vi "TGFrogFINAL.vi"() -> ()   [LabVIEW 2013]
uses:
  <vilib>/Analysis/2dsp.llb/Complex FFT.vi
  <vilib>/Analysis/2dsp.llb/Inverse Complex FFT.vi
  <vilib>/Analysis/NI_AALPro.lvlib
panel:
  out "Error":dbl(graph)
  out "Stationary Solution":bool
  out "Current Error":dbl
  out "Target Error":dbl
  out "size(s) 3":i32
  out "size(s) 2":i32[](array[numeric])
  out "element 2":i32
  in  "Max Iterations":i32
  out "Numeric":i32
  out "element":i32
  out "Experiment Trace":dbl[][](graph)
  out "size(s)":i32[](array[numeric])
  in  "PG Test Data":dbl[][](array[numeric])=array129x256[33024 elements]
  in  "Beta":dbl(slide) scale=-0.01..0.01
  in  "Omega":dbl(slide) scale=0.0..0.5
  in  "Tau":dbl(slide) scale=0.0..100.0
  out "Electric Field":dbl[][](graph)
  out "Recovered Trace":dbl[][](graph)
  out "Gating Visualize":dbl[][](graph)
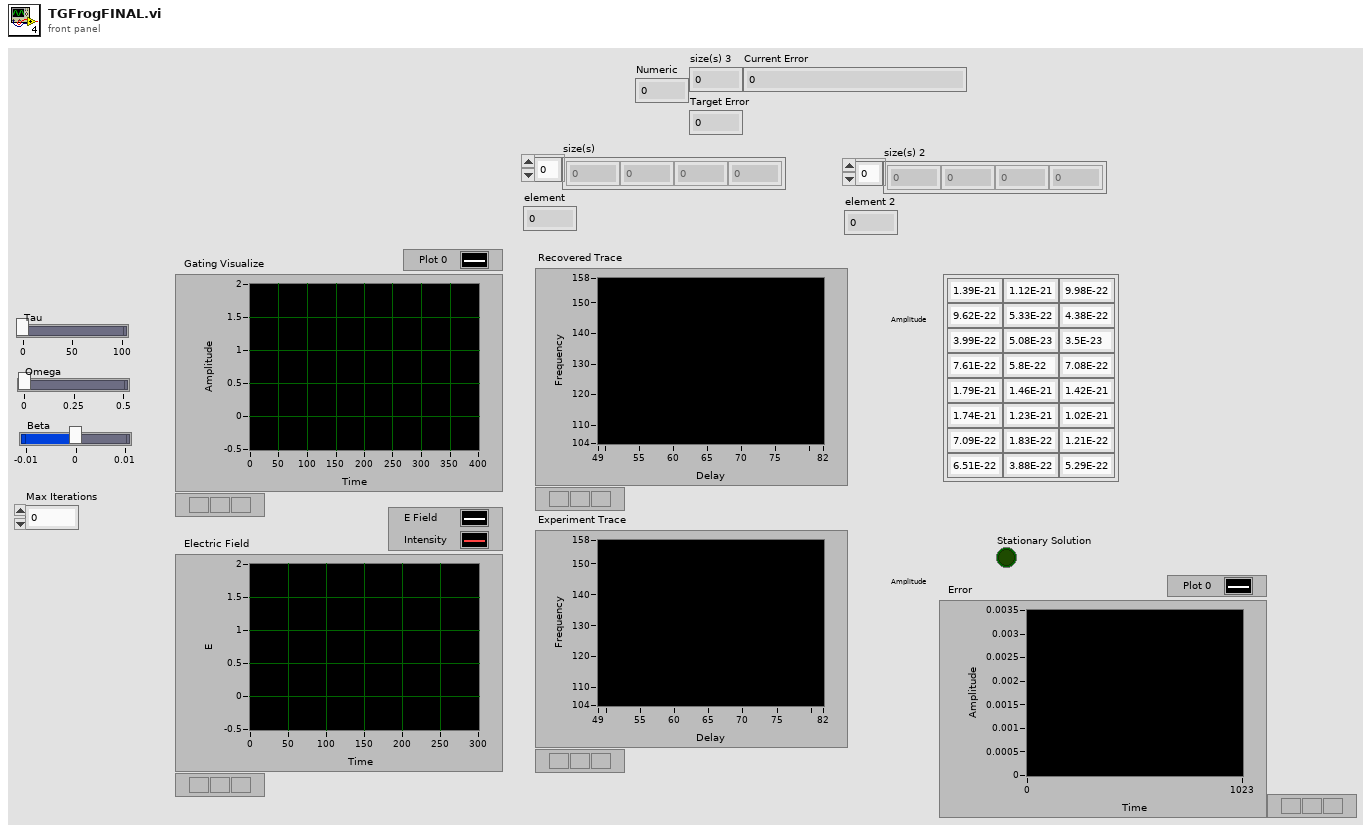
[diagram p1: front panel]
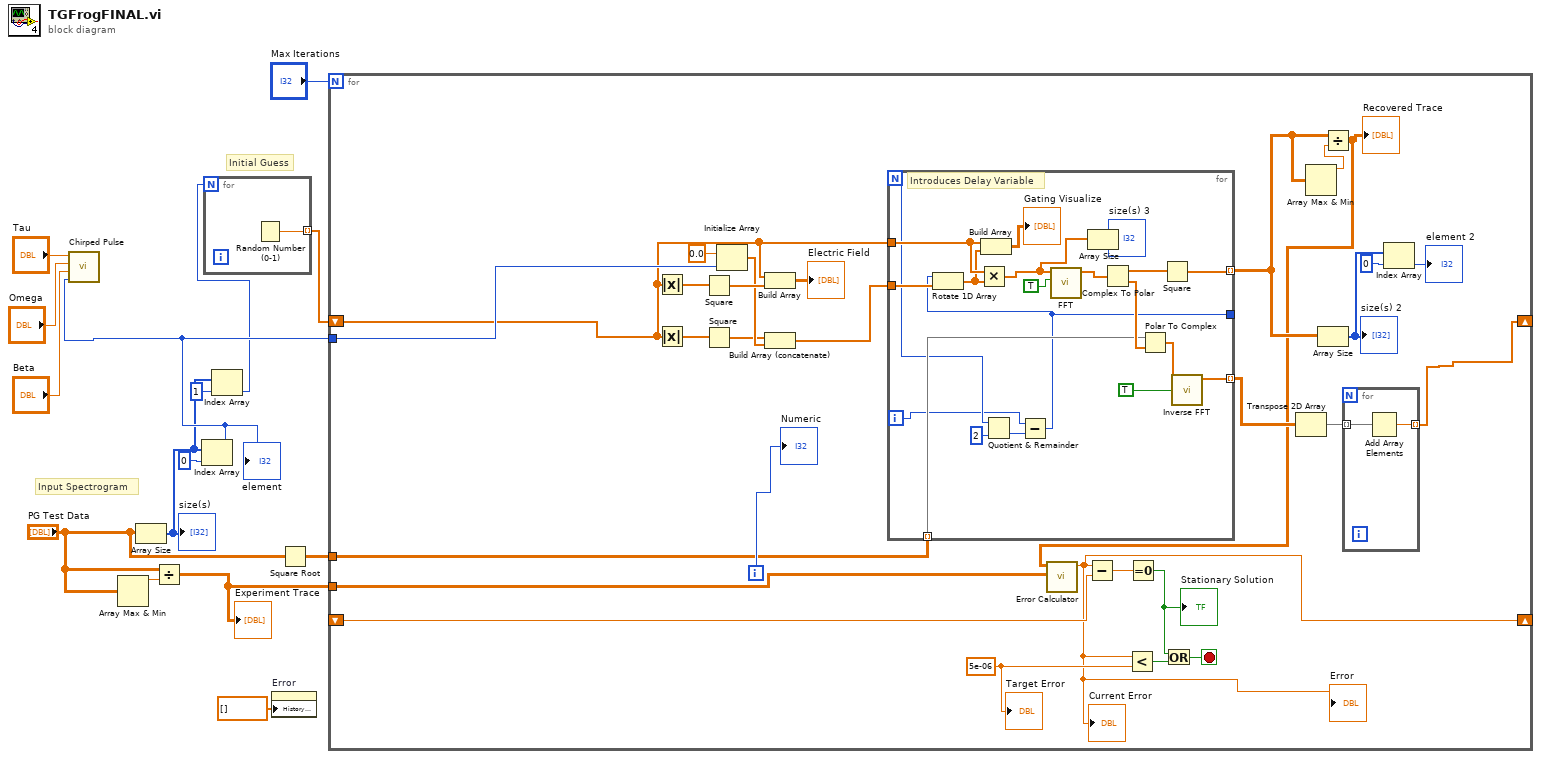
[diagram p0: block diagram]
diagram:
  # "Initial Guess"
  # "Input Spectrogram"
  n1 = Array Max & Min(array="PG Test Data") -> (max value=w7:dbl)  [unwired: 3 out]
  n2 = Array Size(array="PG Test Data") -> (size(s)=w5:i32[])
  "size(s)" <- w5
  n3 = Divide(x="PG Test Data", y=w7) -> (x/y=w2:dbl[][])
  "Experiment Trace" <- w2
  n4 = Index Array(array=w5, index=0) -> (element=w9:i32)
  "element" <- w9
  n5 = call "Chirped Pulse.vi"("Numeric"=w9, "Beta"="Beta", "Omega"="Omega", "Tau"="Tau") -> ()  [unwired: 6 in, 2 out]
  n6 = Index Array(array=w5, index=1) -> (element=w3:i32)
  n7 = for {
    N: w3 -> [_]
    tunnel: [w16] -> w8 mode=indexing
    n8 = Random Number (0-1)() -> (number: 0 to 1=w16:dbl)
  }
  n9 = property on="Error" class="WFChart (strict)"("History Data"=dbl[] []) -> ()  [unwired: 2 in, 2 out]
  n10 = Square Root(x="PG Test Data") -> (sqrt(x)=w10:dbl[][])
  n11 = for {
    N: "Max Iterations" -> [_]
    tunnel: w10 -> [w26]
    tunnel: w9 -> [w37]
    shift-right: [w28] -> _
    shift-left: w8 -> [w30]
    shift-right: [w17] -> _
    shift-left: _ -> [w22]
    tunnel: w2 -> [w19]
    i -> [w45]
    stop <- w24 stop-if-true
    w23 = 5e-06 ("y")
    n12 = Absolute Value(x=w30) -> (abs(x)=w42:dbl[])
    n13 = Absolute Value(x=w30) -> (abs(x)=w39:dbl[])
    n14 = Square(x=w42) -> (x^2=w43:dbl[])
    n15 = Square(x=w39) -> (x^2=w40:dbl[])
    n16 = Initialize Array(0.0 ("element"), w37) -> (w41:dbl[])
    n17 = Build Array(w30, w43) -> (→"Electric Field":cdb[][])
    n18 = Build Array (concatenate)(w40, w41) -> (w29:dbl[])
    n19 = for {
      N -> [w56]
      tunnel: w30 -> [w66]
      tunnel: w29 -> [w67]
      tunnel: [w51] -> w27 mode=indexing
      tunnel: w26 -> [w62] mode=indexing
      tunnel: [w59] -> w32 mode=indexing
      tunnel: [w54] -> _
      i -> [w55]
      # "Introduces Delay Variable"
      n20 = Quotient & Remainder(x=w56, y=2) -> (floor(x/y)=w57:i32)  [unwired: 1 out]
      n21 = Subtract(x=w55, y=w57) -> (x-y=w54:i32)
      n22 = Rotate 1D Array(1:w67, 2:w54) -> (0:w49:dbl[])
      n23 = Multiply(x=w66, y=w49) -> (x*y=w48:cdb[])
      n24 = Build Array(w66, w49) -> (→"Gating Visualize":cdb[][])
      n25 = call-poly <vilib>:"FFT.vi"("shift?"=TRUE, "X"=w48) -> ("FFT {X}"=w53:cdb[])  [unwired: 8 in, 1 out]
      n26 = Array Size(array=w48) -> (size(s)=→"size(s) 3":i32)
      n27 = Complex To Polar(r * e^(i*theta)=w53) -> (r=w64:dbl[], theta=w63:dbl[])
      n28 = Polar To Complex(1:w63, 2:w62) -> (0:w61:cdb[])
      n29 = Square(x=w64) -> (x^2=w51:dbl[])
      n30 = call-poly <vilib>:"Inverse FFT.vi"("shift?"=TRUE, "FFT {X}"=w61) -> ("X"=w59:cdb[])  [unwired: 8 in, 1 out]
    }
    n31 = Transpose 2D Array(2D array=w32) -> (transposed array=w33:cdb[][])
    n32 = Array Max & Min(array=w27) -> (max value=w31:dbl)  [unwired: 3 out]
    n33 = Array Size(array=w27) -> (size(s)=w34:i32[])
    "size(s) 2" <- w34
    n34 = Divide(x=w27, y=w31) -> (x/y=w18:dbl[][])
    "Recovered Trace" <- w18
    n35 = call "Error Calculator.vi"("Recovered Trace"=w18, "Experiment Trace"=w19) -> ("Current Error"=w17:dbl)  [unwired: 8 in]
    "Current Error" <- w17
    "Error" <- w17
    n36 = Subtract(x=w17, y=w22) -> (x-y=w20:dbl)
    n37 = Less?(x=w17, y=w23) -> (x < y?=w25:bool)
    n38 = Equal To 0?(x=w20) -> (x = 0?=w21:bool)
    "Stationary Solution" <- w21
    n39 = Or(x=w21, y=w25) -> (x .or. y?=w24:bool)
    n40 = for {
      tunnel: w33 -> [w46] mode=indexing
      tunnel: [w47] -> w28 mode=indexing
      n41 = Add Array Elements(numeric array=w46) -> (sum=w47:cdb)
    }
    n42 = Index Array(array=w34, index=0) -> (element=→"element 2":i32)
    "Numeric" <- w45
    "Target Error" <- w23
  }
